vi "SH_getShapelet.vi"(8 "error in (no error)":errorcluster, 10 "Index":i32, 11 "ShapeletClass in":refnum<class "Shapelets Search Brute Force.lvclass">) -> (0 "error out":errorcluster, 1 "Shapelet":dbl[][](array[numeric]), 2 "ShapeletForm":cluster{i32[], dbl[]}[](array[cluster]), 3 "ShapeletClass out":refnum<class "Shapelets Search Brute Force.lvclass">, 4 "Fitness":dbl, 5 "ClassLabel":string)   [LabVIEW 2016, in "Shapelets Search (Brute Force).lvlib" / "Shapelets Search Brute Force.lvclass"]
uses:
  Shapelets Search Brute Force.lvclass
  Shapelets Search Brute Force.lvclass/Shapelets Search Brute Force.ctl
panel:
  # "This VI is a part of BCI Design library, http://www.ru-bci.org \nCopyright © 2020, Sotnikov Peter, All rights reserved. License: GNU GPLv3"
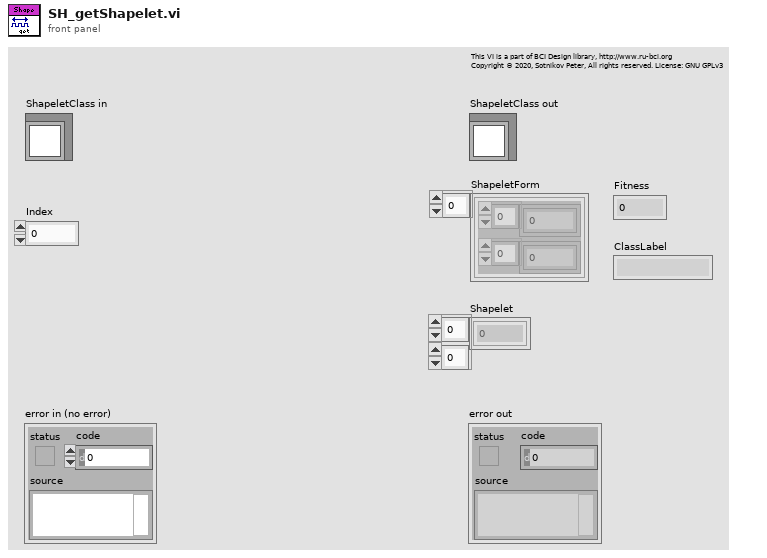
[diagram p1: front panel]
types:
  T1 = cluster{"ClassLabel":string, "FeatureVector":dbl[][]}[]
  T2 = typedef "Shapelets Search (Brute Force).lvlib/SH_Shapelet.ctl" = cluster{"TrialIndex":i32, "Shift (in samples)":i32, "Length (in samples)":i32, "Distances":dbl[], "ClassIndecies":i32[], "Fitness":dbl, "Split Point":dbl}
  T3 = cluster{"ClassLabel":string, "FeatureVector":dbl[][]}
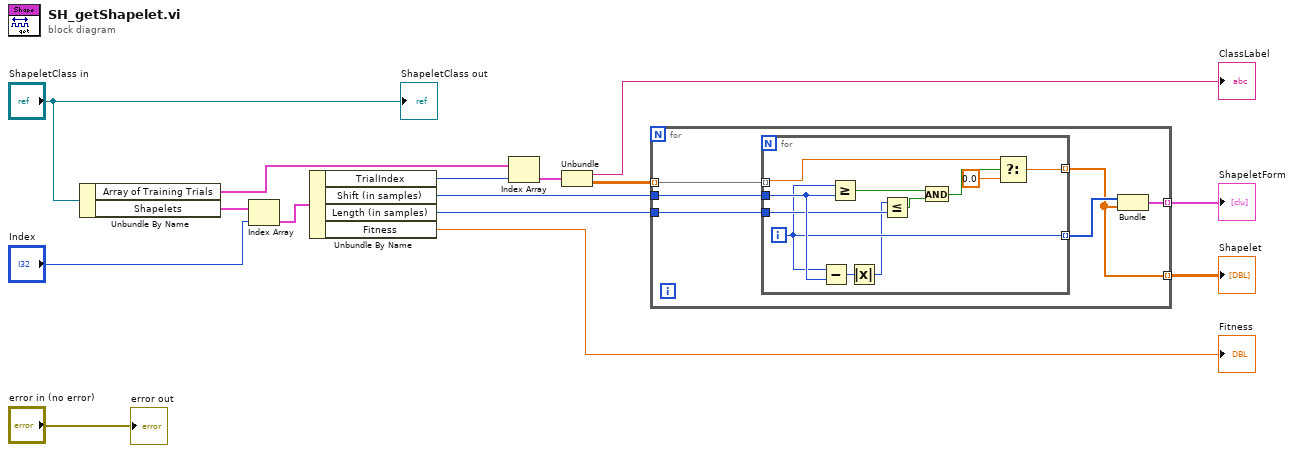
[diagram p0: block diagram]
diagram:
  n1 = Unbundle By Name("ShapeletClass in") -> ("Array of Training Trials"=w11:T1, "Shapelets"=w14:T2[])
  n2 = Index Array(array=w14, index="Index") -> (element=w12:T2)
  n3 = Unbundle By Name(w12) -> ("TrialIndex"=w10:i32, "Shift (in samples)"=w7:i32, "Length (in samples)"=w6:i32, "Fitness"=→"Fitness":dbl)
  n4 = Index Array(array=w11, index=w10) -> (element=w9:T3)
  n5 = Unbundle(w9) -> ("ClassLabel"=→"ClassLabel":string, "FeatureVector"=w8:dbl[][])
  n6 = for {
    tunnel: w8 -> [w16] mode=indexing
    tunnel: w7 -> [w21]
    tunnel: w6 -> [w20]
    tunnel: [w18] -> w4 mode=indexing
    tunnel: [w17] -> w2 mode=indexing
    n7 = for {
      tunnel: w16 -> [w23] mode=indexing
      tunnel: w21 -> [w32]
      tunnel: w20 -> [w31]
      tunnel: [w22] -> w17 mode=indexing
      tunnel: [w26] -> w19 mode=indexing
      i -> [w26]
      n8 = Subtract(x=w26, y=w32) -> (x-y=w25:i32)
      n9 = Greater Or Equal?(x=w26, y=w32) -> (x >= y?=w30:bool)
      n10 = Absolute Value(x=w25) -> (abs(x)=w24:i32)
      n11 = Less Or Equal?(x=w24, y=w31) -> (x <= y?=w29:bool)
      n12 = And(x=w30, y=w29) -> (x .and. y?=w28:bool)
      n13 = Select(t=w23, s=w28, f=0.0) -> (s? t:f=w22:dbl)
    }
    n14 = Bundle(w19, w17) -> (w18:cluster{i32[], dbl[]})  [unwired: 1 in]
  }
  "ShapeletForm" <- w4
  "Shapelet" <- w2
  "error out" <- "error in (no error)"
  "ShapeletClass out" <- "ShapeletClass in"
